vi "Choose View Type.vi"(8 "error in (no error)":errorcluster, 11 "Example Controller Actor in":refnum<class "Example Controller.lvclass">) -> (0 "error out":errorcluster, 3 "Example Controller Actor out":refnum<class "Example Controller.lvclass">)   [LabVIEW 2023, in "Example GUI View.lvlib" / "Example Controller.lvclass"]
uses:
  Example Controller.lvclass
  Example GUI View/Example GUI View.lvclass
  Example Controller.lvclass/Example Controller.ctl
  GUI Views/GUI View/GUI View.lvclass/GUI View.ctl
  Example Controller/Example Controller/Example Controller.lvclass/Example Controller.ctl
  GUI Views/GUI View/properties/Write Container Enqueuer.vi
  Example Controller/Example Controller/properties/Write View Type.vi
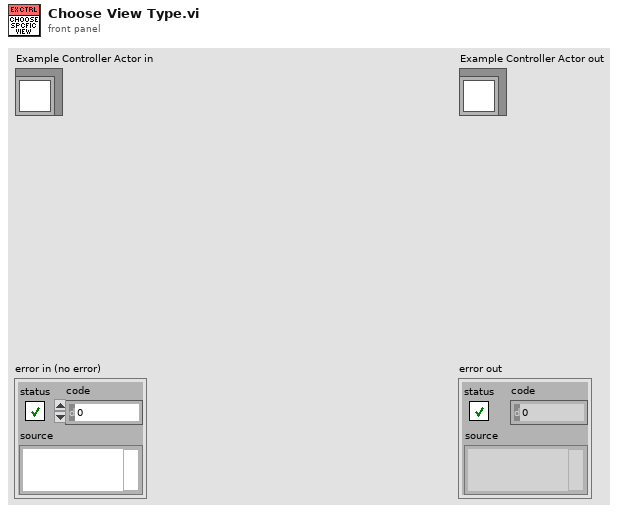
[diagram p1: front panel]
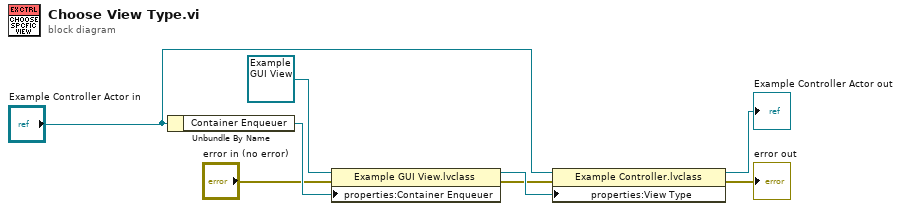
[diagram p0: block diagram]
diagram:
  n1 = Unbundle By Name("Example Controller Actor in") -> ("Container Enqueuer"=w3:refnum<class "Message Enqueuer.lvclass">)
  n2 = property class="Example GUI View.lvclass"(reference=refnum<class "Example GUI View.lvclass"> refnum ("Example GUI View Actor.lvlib:Example GUI View Actor.lvclass"), error in="error in (no error)", "properties:Container Enqueuer"=w3) -> (reference out=w5:refnum<class "Example GUI View.lvclass">, error out=w1:errorcluster)
  n3 = property class="Example Controller.lvclass"(reference="Example Controller Actor in", error in=w1, "properties:View Type"=w5) -> (reference out=→"Example Controller Actor out":refnum<class "Example Controller.lvclass">, error out=→"error out":errorcluster)
